vi "Call VI.vi"(4 "output info":T1[](array[typedef]), 6 "input info":T2[](array[typedef]), 8 "error in (no error)":errorcluster, 9 "Input Values":string[](array[string]), 10 "Input Names":string[](array[string]), 11 "VI in":refnum<vi>) -> (0 "error out":errorcluster, 1 "output values":string[](array[string]), 2 "output names":string[](array[string]), 3 "pictures":string[](array[string]))   [LabVIEW 2020, in "MCP Server.lvlib"]
uses:
  MCP Server.lvlib
  Input Parameter.ctl
  Output Parameter.ctl
  e41d13a5-b533-4b14-93c6-4ba0c6d1a2bf.vi
  b3e15f38-d5ce-4610-9e48-04c139622bf1.vi
  b8448edb-b4b5-47d7-90b3-aea56ff88df2.vi
  989a8bd6-30de-4821-a40a-8a1d239f579d.vi
  8b9ff06f-0ef6-44a3-acf4-59db1b6b1b31.vi
  0616d323-15ae-486a-97f1-8f6250f713f5.vi
  9d91f7f2-9bb6-4ecb-af38-d838d0deb514.vi
  fd11c23e-f9de-4047-abc2-5cee66b205fd.vi
  1521ffbb-a9e1-42f7-9593-99dcb95d3f2d.vi
  522b1827-3836-432c-b8b2-8f0c55f6feb7.vi
  4c506424-2eda-4aef-885b-07ff0af22ab5.vi
  4168f984-ecba-4b3e-98aa-6b303e1fc845.vi
  <vilib>/JDP Science/JSONtext/JSON text to Variant.vi
  <vilib>/JDP Science/JSONtext/Variant to JSON Text.vi
  <vilib>/JDP Science/JSONtext/LVClass Serializer/JSONtext LVClass Serializer.lvclass
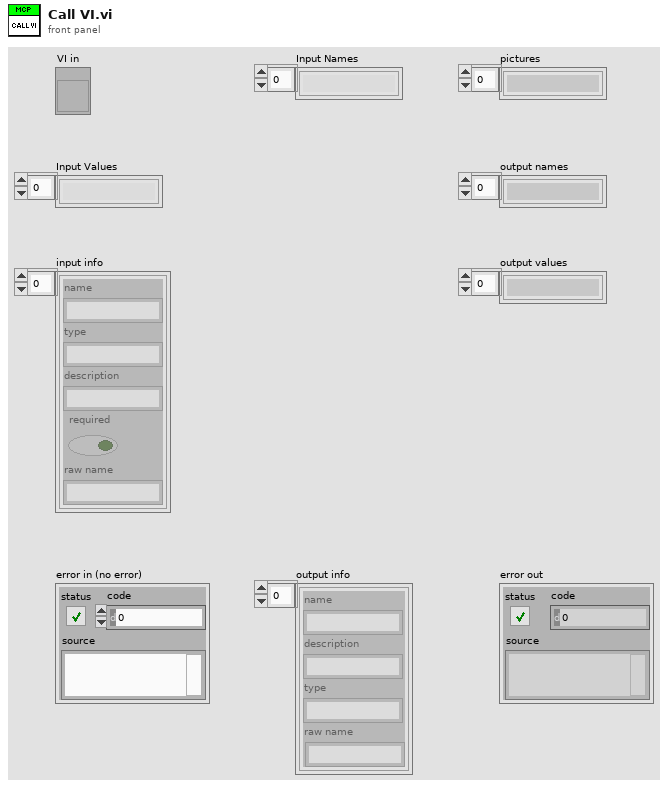
[diagram p1: front panel]
types:
  T1 = typedef "MCP Server.lvlib/Output Parameter.ctl" = cluster{"name":string, "description":string, "type":string, "raw name":string}
  T2 = typedef "MCP Server.lvlib/Input Parameter.ctl" = cluster{"name":string, "type":string, "description":string, "required":bool, "raw name":string}
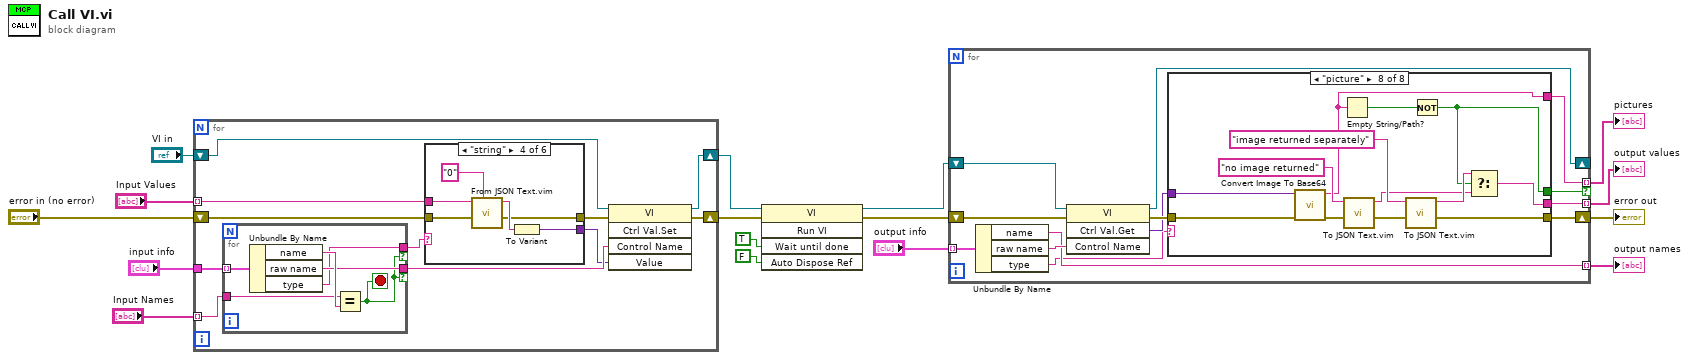
[diagram p0: block diagram]
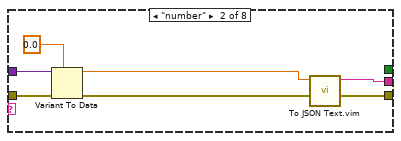
[diagram p3: hidden frame]
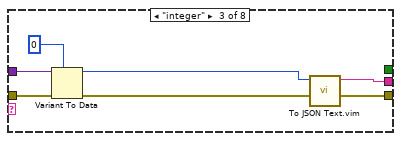
[diagram p4: hidden frame]
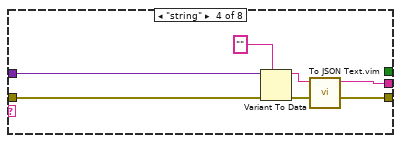
[diagram p5: hidden frame]
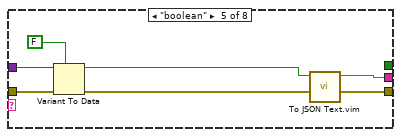
[diagram p6: hidden frame]
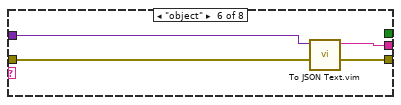
[diagram p7: hidden frame]
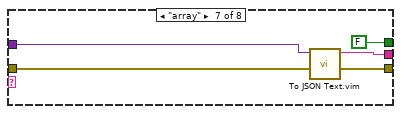
[diagram p8: hidden frame]
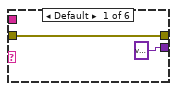
[diagram p9: hidden frame]
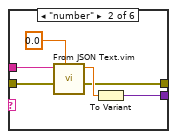
[diagram p10: hidden frame]
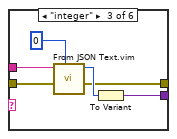
[diagram p11: hidden frame]
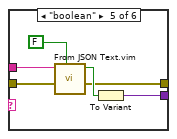
[diagram p12: hidden frame]
diagram:
  n1 = for {
    tunnel: "Input Values" -> [w21] mode=indexing
    tunnel: "Input Names" -> [w23] mode=indexing
    shift-right: [w26] -> w3
    shift-left: "VI in" -> [w27]
    shift-right: [w25] -> w4
    shift-left: "error in (no error)" -> [w18]
    tunnel: "input info" -> [w24]
    n2 = for {
      tunnel: w24 -> [w61] mode=indexing
      tunnel: w23 -> [w59]
      tunnel: [w58] -> w22 if=w56
      tunnel: [w57] -> w19 if=w56
      stop <- w56 stop-if-true
      n3 = Unbundle By Name(w61) -> ("name"=w60:string, "raw name"=w58:string, "type"=w57:string)
      n4 = Equal?(x=w59, y=w60) -> (x = y?=w56:bool)
    }
    n5 = case shown="\"string\"" w19 {
      tunnel: w21 -> [_ w35 w41 w47 w53 w55]
      tunnel: [variant ("Variant") w33 w39 w45 w51 w55] -> w20
      tunnel: w18 -> [w28 w31 w36 w43 w49 w54]
      tunnel: [w28 w30 w37 w42 w48 w54] -> w17
      frame Default {
      }
      frame "number" {
        n6 = call "From JSON Text.vim"("Data Type and Default Value"=0.0, "error in (no error)"=w31, "JSON"=w35) -> ("error out"=w30:errorcluster, "Data out"=w34:dbl)  [unwired: 7 in]
        n7 = To Variant(anything=w34) -> (Variant=w33:variant)
      }
      frame "integer" {
        n8 = call "From JSON Text.vim"("Data Type and Default Value"=i64 0, "error in (no error)"=w36, "JSON"=w41) -> ("error out"=w37:errorcluster, "Data out"=w40:i64)  [unwired: 7 in]
        n9 = To Variant(anything=w40) -> (Variant=w39:variant)
      }
      frame "string" {
        n10 = call "From JSON Text.vim"("Data Type and Default Value"="0", "error in (no error)"=w43, "JSON"=w47) -> ("error out"=w42:errorcluster, "Data out"=w46:string)  [unwired: 7 in]
        n11 = To Variant(anything=w46) -> (Variant=w45:variant)
      }
      frame "boolean" {
        n12 = call "From JSON Text.vim"("Data Type and Default Value"=FALSE, "error in (no error)"=w49, "JSON"=w53) -> ("error out"=w48:errorcluster, "Data out"=w52:bool)  [unwired: 7 in]
        n13 = To Variant(anything=w52) -> (Variant=w51:variant)
      }
      frame "object" {
      }
    }
    n14 = invoke class="VI" method="Ctrl Val.Set"(reference=w27, error in=w17, "Control Name"=w22, "Value"=w20) -> (reference out=w26:refnum<vi>, error out=w25:errorcluster)  [unwired: 1 in, 3 out]
  }
  n15 = invoke class="VI" method="Run VI"(reference=w3, error in=w4, "Wait until done"=TRUE ("Wait Until Done"), "Auto Dispose Ref"=FALSE ("Auto Dispose Reference")) -> (reference out=w7:refnum<vi>, error out=w8:errorcluster)  [unwired: 1 in, 3 out]
  n16 = for {
    shift-right: [w73] -> _
    shift-left: w7 -> [w74]
    shift-right: [w66] -> w15
    shift-left: w8 -> [w71]
    tunnel: "output info" -> [w70] mode=indexing
    tunnel: [w67] -> w11 mode=indexing
    tunnel: [w65] -> w10 mode=indexing
    tunnel: [w63] -> w13 mode=indexing if=w62
    n17 = Unbundle By Name(w70) -> ("name"=w67:string, "raw name"=w68:string, "type"=w64:string)
    n18 = invoke class="VI" method="Ctrl Val.Get"(reference=w74, error in=w71, "Control Name"=w68) -> (reference out=w73:refnum<vi>, error out=w72:errorcluster, "Get Control Value Variant"=w69:variant)  [unwired: 1 in, 1 out]
    n19 = case shown="\"picture\"" w64 {
      tunnel: w72 -> [w75 w82 w89 w96 w103 w107 w112 w124]
      tunnel: w69 -> [_ w78 w85 w92 w99 w104 w108 w125]
      tunnel: [w75 w81 w88 w95 w102 w106 w111 w121] -> w66
      tunnel: [_ w80 w87 w94 w101 w105 w109 w118] -> w65
      tunnel: [_ _ _ _ _ _ _ w119] -> w63
      tunnel: [_ _ _ _ _ _ FALSE w115] -> w62
      frame Default {
      }
      frame "number" {
        n20 = Variant To Data(error in=w82, type=0.0, Variant=w78) -> (data=w76:dbl, error out=w79:errorcluster)
        n21 = call "To JSON Text.vim"("error in (no error)"=w79, "Anything"=w76) -> ("error out"=w81:errorcluster, "<JSON>"=w80:string)  [unwired: 8 in]
      }
      frame "integer" {
        n22 = Variant To Data(error in=w89, type=i64 0, Variant=w85) -> (data=w83:i64, error out=w86:errorcluster)
        n23 = call "To JSON Text.vim"("error in (no error)"=w86, "Anything"=w83) -> ("error out"=w88:errorcluster, "<JSON>"=w87:string)  [unwired: 8 in]
      }
      frame "string" {
        n24 = Variant To Data(error in=w96, type="", Variant=w92) -> (data=w90:string, error out=w93:errorcluster)
        n25 = call "To JSON Text.vim"("error in (no error)"=w93, "Anything"=w90) -> ("error out"=w95:errorcluster, "<JSON>"=w94:string)  [unwired: 8 in]
      }
      frame "boolean" {
        n26 = Variant To Data(error in=w103, type=FALSE, Variant=w99) -> (data=w97:bool, error out=w100:errorcluster)
        n27 = call "To JSON Text.vim"("error in (no error)"=w100, "Anything"=w97) -> ("error out"=w102:errorcluster, "<JSON>"=w101:string)  [unwired: 8 in]
      }
      frame "object" {
        n28 = call "To JSON Text.vim"("error in (no error)"=w107, "Anything"=w104) -> ("error out"=w106:errorcluster, "<JSON>"=w105:string)  [unwired: 8 in]
      }
      frame "array" {
        n29 = call "To JSON Text.vim"("error in (no error)"=w112, "Anything"=w108) -> ("error out"=w111:errorcluster, "<JSON>"=w109:string)  [unwired: 8 in]
      }
      frame "picture" {
        n30 = call "Convert Image To Base64.vi"("error in (no error)"=w124, "Get Control Value Variant"=w125) -> ("error out"=w114:errorcluster, "<JSON>"=w119:string)  [unwired: 8 in]
        n31 = Empty String/Path?(string/path=w119) -> (empty?=w116:bool)
        n32 = call "To JSON Text.vim"("error in (no error)"=w114, "Anything"="no image returned" ("<JSON>")) -> ("error out"=w113:errorcluster, "<JSON>"=w117:string)  [unwired: 8 in]
        n33 = call "To JSON Text.vim"("error in (no error)"=w113, "Anything"="image returned separately" ("<JSON>")) -> ("error out"=w121:errorcluster, "<JSON>"=w122:string)  [unwired: 8 in]
        n34 = Not(x=w116) -> (.not. x?=w115:bool)
        n35 = Select(t=w122, s=w115, f=w117) -> (s? t:f=w118:string)
      }
    }
  }
  "error out" <- w15
  "pictures" <- w13
  "output names" <- w11
  "output values" <- w10
